vi "Emi Cmd3.vi"(0 "X-CAN en entrée":refnum<class "X-CAN.lvclass">, 1 "Numéro Image Attente":u8[](array[numeric]), 2 "Num Img Proc":u8[](array[numeric]), 3 "Durée Img Proc":u8[](array[numeric]), 4 "Durée process":u8[](array[numeric]), 5 "entrée d'erreur (pas d'erreur)":errorcluster, 7 "Num Emi In":u8, 8 "Emission":bool) -> (13 "Num Emi  Out":u8, 14 "X-CAN en sortie":refnum<class "X-CAN.lvclass">, 19 "sortie d'erreur":errorcluster)   [LabVIEW 2014]
uses:
  <vilib>/Stratom, Inc/X-CAN for myRIO (API)/X-CAN Class/X-CAN.lvclass
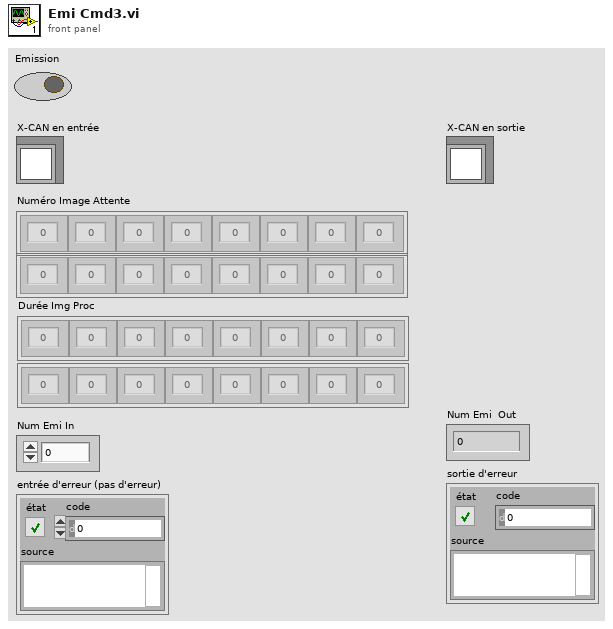
[diagram p1: front panel]
types:
  T1 = cluster{i32, bool, bool, "Numéro Image Attente ":u8[], "seconds since 1Jan1904":timestamp}
  T2 = cluster{i32, bool, bool, "Num Img Proc":u8[], "seconds since 1Jan1904":timestamp}
  T3 = cluster{i32, bool, bool, "Durée Img Proc  ":u8[], "seconds since 1Jan1904":timestamp}
  T4 = cluster{i32, bool, bool, "Durée process":u8[], "seconds since 1Jan1904":timestamp}
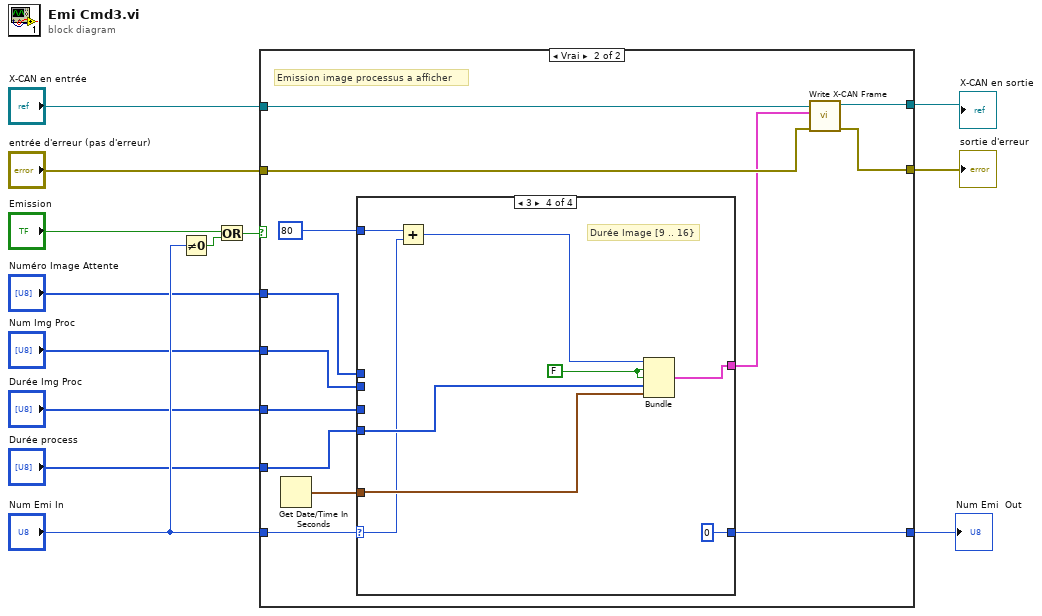
[diagram p0: block diagram]
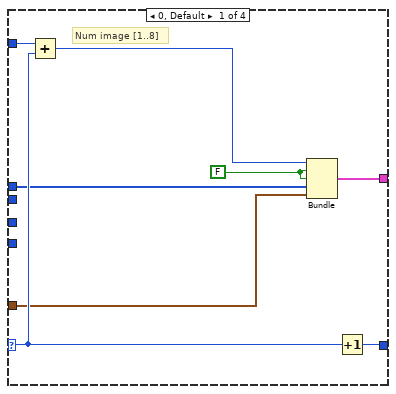
[diagram p3: hidden frame]
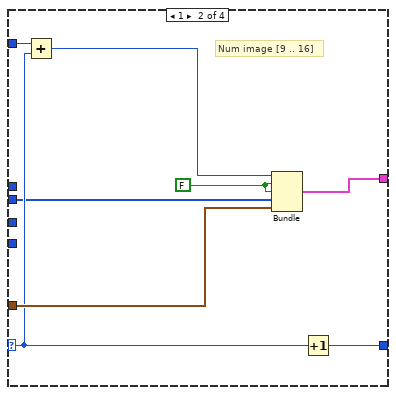
[diagram p4: hidden frame]
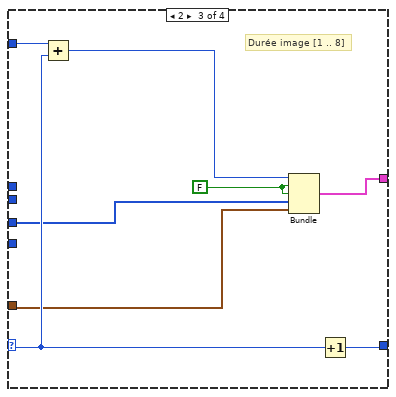
[diagram p5: hidden frame]
diagram:
  n1 = Not Equal To 0?(x="Num Emi In") -> (x != 0?=w7:bool)
  n2 = Or(x="Emission", y=w7) -> (x .or. y?=w9:bool)
  n3 = case shown="Vrai" w9 {
    tunnel: [w15 w29] -> w13
    tunnel: "entrée d'erreur (pas d'erreur)" -> [w15 w28]
    tunnel: [w16 w27] -> w11
    tunnel: "X-CAN en entrée" -> [w16 w26]
    tunnel: "Num Emi In" -> [w14 w23]
    tunnel: [w14 w22] -> w5
    tunnel: "Numéro Image Attente" -> [_ w21]
    tunnel: "Num Img Proc" -> [_ w19]
    tunnel: "Durée Img Proc" -> [_ w18]
    tunnel: "Durée process" -> [_ w17]
    frame False {
    }
    frame True {
      # "Emission image processus a afficher"
      n4 = Get Date/Time In Seconds() -> (seconds since 1Jan1904=w25:timestamp)
      n5 = case shown="3" w23 {
        selector: w23 -> [w34 w41 w50 w56]
        tunnel: w25 -> [w31 w45 w48 w58]
        tunnel: 80 -> [w35 w42 w51 w59]
        tunnel: [w36 w43 w46 0] -> w22
        tunnel: w21 -> [w32 _ _ _]
        tunnel: [w30 w38 w47 w54] -> w20
        tunnel: w19 -> [_ w39 _ _]
        tunnel: w18 -> [_ _ w49 _]
        tunnel: w17 -> [_ _ _ w57]
        frame 0, Default {
          w37 = FALSE
          # "Num image [1..8]"
          n6 = Add(x=w35, y=w34) -> (x+y=w33:i32)
          n7 = Bundle(w33, w37, w37, "Numéro Image Attente"=w32, "seconds since 1Jan1904"=w31) -> (w30:T1)  [unwired: 1 in]
          n8 = Increment(x=w34) -> (x+1=w36:u8)
        }
        frame 1 {
          w44 = FALSE
          # "Num image [9 .. 16]"
          n9 = Add(x=w42, y=w41) -> (x+y=w40:i32)
          n10 = Bundle(w40, w44, w44, "Num Img Proc"=w39, "seconds since 1Jan1904"=w45) -> (w38:T2)  [unwired: 1 in]
          n11 = Increment(x=w41) -> (x+1=w43:u8)
        }
        frame 2 {
          w53 = FALSE
          # "Durée image [1 .. 8]"
          n12 = Add(x=w51, y=w50) -> (x+y=w52:i32)
          n13 = Bundle(w52, w53, w53, "Durée Img Proc"=w49, "seconds since 1Jan1904"=w48) -> (w47:T3)  [unwired: 1 in]
          n14 = Increment(x=w50) -> (x+1=w46:u8)
        }
        frame 3 {
          w61 = FALSE
          # "Durée Image [9 .. 16}"
          n15 = Add(x=w59, y=w56) -> (x+y=w60:i32)
          n16 = Bundle(w60, w61, w61, "Durée process"=w57, "seconds since 1Jan1904"=w58) -> (w54:T4)  [unwired: 1 in]
        }
      }
      n17 = call <vilib>:"Write X-CAN Frame.vi"("error in"=w28, "CAN Frame"=w20, "X-CAN Session in"=w26) -> ("error out"=w29:errorcluster, "X-CAN Session out"=w27:refnum<class "X-CAN.lvclass">)  [unwired: 7 in]
    }
  }
  "sortie d'erreur" <- w13
  "X-CAN en sortie" <- w11
  "Num Emi  Out" <- w5
